vi "Excel Open Worksheet.vi"(0 "Sheets Ref In":refnum<k7>, 7 "Sheet#":i32, 11 "Error In":errorcluster) -> (4 "Sheets Ref Out":refnum<k7>, 8 "Worksheet Ref Out":refnum<k7>, 10 "Error Out":errorcluster, 15 "Cells Ref Out":refnum<k7>)   [LabVIEW 2019]
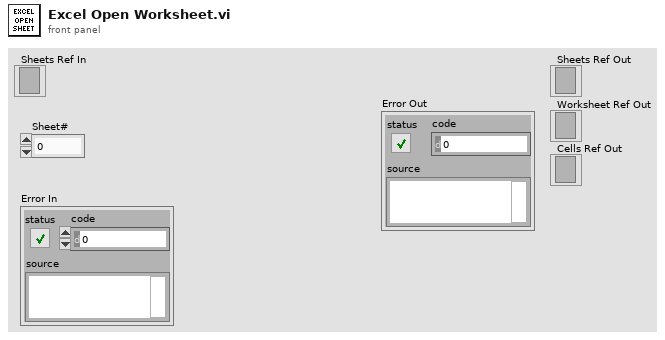
[diagram p1: front panel]
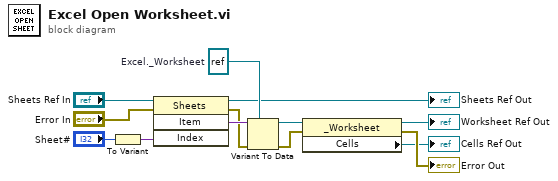
[diagram p0: block diagram]
diagram:
  w6 = refnum<k7> refnum  # Excel._Worksheet
  n1 = To Variant(anything="Sheet#") -> (Variant=w10:variant)
  n2 = invoke class="Sheets" method="Item"(reference="Sheets Ref In", error in="Error In", "Index"=w10) -> (reference out=→"Sheets Ref Out":refnum<k7>, error out=w9:errorcluster, "Item"=w11:variant)  [unwired: 1 in, 1 out]
  n3 = Variant To Data(error in=w9, type=w6, Variant=w11) -> (data=w7:refnum<k7>, error out=w8:errorcluster)
  n4 = property class="_Worksheet"(reference=w7, error in=w8) -> (reference out=→"Worksheet Ref Out":refnum<k7>, error out=→"Error Out":errorcluster, "Cells"=→"Cells Ref Out":refnum<k7>)
